vi "LabVIEWArduinoModbus2.vi"() -> ()   [LabVIEW 2014]
uses:
  <vilib>/Modbus/master/Create Master Instance (Serial).vi
  <vilib>/Modbus/master/Modbus Master.lvclass
panel:
  out "波形图表":u16[](graph)
  in  "停止按钮":bool
  out "error out":errorcluster caption="错误输出"
  in  "coil value":bool caption="线圈值"
  in  "address":u16=13 caption="地址"
  in  "error in (no error)":errorcluster caption="错误输入（无错误）"
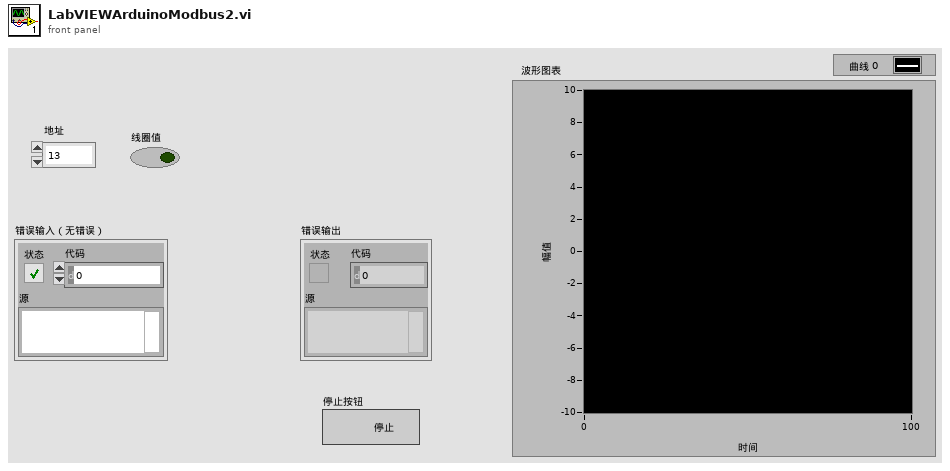
[diagram p1: front panel]
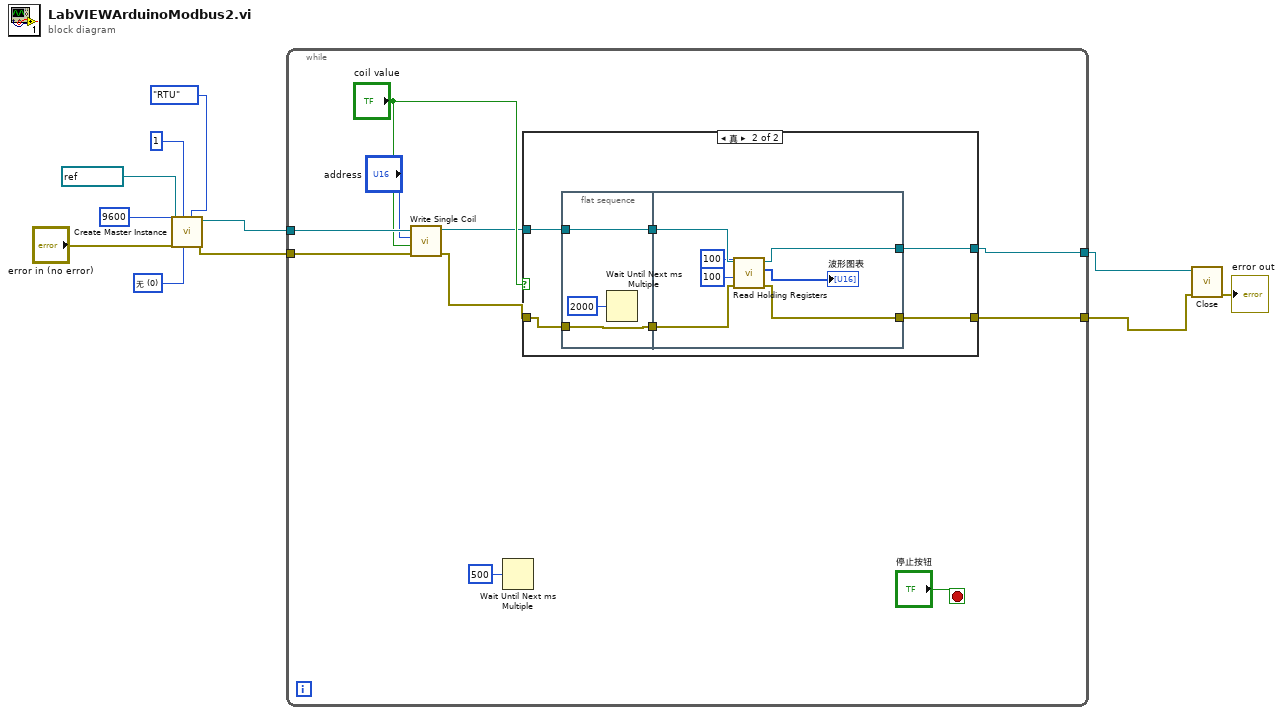
[diagram p0: block diagram]
diagram:
  w7 = u16 0 items=["无", "奇", "偶"] ("parity (Even)")
  n1 = call-poly <vilib>:"Create Master Instance.vi"("serial type"=enum16{"RTU", "ASCII"}."RTU", "parity (Even)"=w7, "unit ID"=u8 1, "error in (no error)"="error in (no error)", "baud rate (9600)"=u32 9600, "VISA resource name"=refnum<visa-resource-name> "COM3") -> ("error out"=w5:errorcluster, "serial master instance"=w6:refnum<class "Modbus Master.lvclass">)  [unwired: 4 in]
  n2 = while {
    tunnel: w6 -> [w21]
    tunnel: w5 -> [w19]
    tunnel: [w14] -> w2
    tunnel: [w12] -> w1
    stop <- "停止按钮" stop-if-true
    n3 = call-dynamic "Write Single Coil.vi"("error in (no error)"=w19, "coil value"="coil value", "address"="address", "Modbus master in"=w21) -> ("error out"=w13:errorcluster, "Modbus master out"=w15:refnum<class "Modbus Master.lvclass">)  [unwired: 6 in]
    n4 = Wait Until Next ms Multiple(millisecond multiple=u32 500 ("毫秒倍数")) -> ()  [unwired: 1 out]
    n5 = case shown="真" "coil value" {
      tunnel: w15 -> [w23 w29]
      tunnel: [w23 w25] -> w14
      tunnel: w13 -> [w22 w27]
      tunnel: [w22 w24] -> w12
      frame False {
      }
      frame True {
        n6 = flat-sequence {
          tunnel: w29 -> [w31]
          tunnel: [w31] -> w28
          tunnel: w27 -> [w30]
          tunnel: [w30] -> w26
          tunnel: w28 -> [w39]
          tunnel: w26 -> [w38]
          tunnel: [w35] -> w25
          tunnel: [w34] -> w24
          frame #0 {
            n7 = Wait Until Next ms Multiple(millisecond multiple=u32 2000 ("毫秒倍数")) -> ()  [unwired: 1 out]
          }
          frame #1 {
            n8 = call-dynamic "Read Holding Registers.vi"("error in (no error)"=w38, "number of holding registers"=u16 100, "starting address"=u16 100, "Modbus master in"=w39) -> ("error out"=w34:errorcluster, "register values"=→"波形图表":u16[], "Modbus master out"=w35:refnum<class "Modbus Master.lvclass">)  [unwired: 5 in]
          }
        }
      }
    }
  }
  n9 = call-dynamic "Close.vi"("error in (no error)"=w1, "Modbus master in"=w2) -> ("error out"=→"error out":errorcluster)  [unwired: 9 in]
